vi "HFRR ADV v017 new software.vi"() -> ()   [LabVIEW 2025] (continued)
          tunnel: [w1639] -> w1630
          tunnel: [w1638] -> w1631
          tunnel: w1627 -> [w1637]
          tunnel: w1626 -> [w1636]
          stop <- TRUE stop-if-true
          n1455 = property class="Instr" props=["Serial Settings:Number of Bytes at Serial Port"](reference=w1636, error in=w1637) -> (reference out=w1641:refnum<visa-resource-name>, error out=w1640:errorcluster)  [unwired: 1 out]
          n1456 = VISA Read(VISA resource name=w1641, byte count=u32 50, error in (no error)=w1640) -> (VISA resource name out=w1638:refnum<visa-resource-name>, read buffer=→"UNI READ":string, error out=w1639:errorcluster)  [unwired: 1 out]
          n1457 = Wait (ms)(milliseconds to wait=u32 5) -> ()  [unwired: 1 out]
        }
      }
      frame Error {
        w1656 = u16 0 items=["None", "XON/XOFF", "RTS/CTS", "XON/XOFF & RTS/CTS", "DTR/DSR", "XON/XOFF & DTR/DSR"] ("flow control (0:none)  2")
        w1654 = u16 10 items=["1.0"=10, "1.5"=15, "2.0"=20] ("stop bits 2")
        w1652 = u16 0 items=["None", "Odd", "Even", "Mark", "Space"] ("parity 2")
        w1653 = u32 10000  # timeout (10sec)
        n1458 = VISA Close(VISA resource name=w1648, error in (no error)=w1646) -> (error out=w1649:errorcluster)
        n1459 = local write "Port 1a"(FALSE ("Port 1a")) -> ()
        n1460 = local read "Com Port 1"() -> (w1643:refnum<visa-resource-name>)
        n1461 = call <vilib>:"Clear Errors.vi"("error in (no error)"=w1649) -> ("error out"=w1647:errorcluster)  [unwired: 5 in, 1 out]
        n1462 = call-poly "VISA Configure Serial Port"("VISA resource name"=w1643, "timeout (10sec)"=w1653, "baud rate (9600)"=u32 250000 ("baud rate  2"), "data bits (8)"=u16 8 ("data bits  2"), "parity (0:none)"=w1652, "error in (no error)"=w1647, "stop bits (10: 1 bit)"=w1654, "flow control (0:none)"=w1656) -> ("VISA resource name out"=w1657:refnum<visa-resource-name>, "error out"=w1658:errorcluster)  [unwired: 6 in]
        n1463 = flat-sequence {
          tunnel: w1657 -> [w1660]
          tunnel: w1658 -> [w1659]
          tunnel: [w1660] -> w1650
          tunnel: [w1659] -> w1644
          frame #0 {
            n1464 = Wait (ms)(milliseconds to wait=u32 50) -> ()  [unwired: 1 out]
          }
        }
        "Residual Uno" <- ""
        "Port 1 Error" <- w1644
      }
    }
    n1465 = local read "Quit"() -> (w1605:bool)
    "Error Uno" <- w1610
  }
  n1466 = while {
    stop <- w1671 stop-if-true
    # "V0OLTAGE TO STROKE (peice vise calibration)"
    n1467 = local read "LVDT MIN"() -> (w1662:dbl)
    n1468 = Wait (ms)(milliseconds to wait=u32 10) -> ()  [unwired: 1 out]
    n1469 = local read "LVDT Peak"() -> (w1663:dbl)
    n1470 = formula code="// Dynamic Parameterized Linear Interpolation Node\n// Inputs: vpp_val, voltages (Array), distances (Array)\n// Outputs: stroke\n\nint i = 0;\nint segments = 11; // 12 points make 11 interpolation segments\n\n// 1. Lower Boundary Clamp\nif (vpp_val <= voltages[0]) {\n    stroke = distances[0];\n}\n// 2. Upper Boundary Clamp\nelse if (vpp_val >= voltages[segments]) {\n    stroke = distances[segments];\n}\n// 3. Dynamic Segment Search Loop\nelse {\n    stroke = distances[0]; // Fallback baseline\n    for (i = 0; i < segments; i++) {\n        if (vpp_val >= voltages[i] && vpp_val <= voltages[i+1]) {\n            // Standard linear interpolation formula using array lookups\n            stroke = distances[i] + (vpp_val - voltages[i]) * (distances[i+1] - distances[i]) / (voltages[i+1] - voltages[i]);\n            break; // Segment found, safely exit the loop\n        }\n    }\n}"("vpp_val"=w1663, "voltages"="calibration values", "distances"="STROKE") -> ("stroke"=→"LVDT STROKE":dbl)
    n1471 = local read "Calibration Tare Value"() -> (w1667:dbl)
    n1472 = local read "Calibration Tare"() -> (w1665:bool)
    n1473 = Subtract(x=w1662, y=w1667) -> (x-y=→"LVDT STROKE  Calibration":dbl)
    n1474 = case shown="True" w1665 {
      selector: w1665 -> [_ w1673]
      tunnel: w1662 -> [_ w1674]
      frame False {
      }
      frame True {
        n1475 = Not(x=w1673) -> (.not. x?=w1672:bool)
        n1476 = local write "Calibration Tare"(w1672) -> ()
        "Calibration Tare Value" <- w1674
      }
    }
    n1477 = local read "Quit"() -> (w1671:bool)
  }
  n1478 = while {
    stop <- w1694 stop-if-true
    n1479 = call <vilib>:"High Resolution Polling Wait.vi"("seconds to wait"=0.02) -> ()  [unwired: 10 in, 1 out]
    n1480 = local read "Due read"() -> (w1692:string)
    n1481 = Spreadsheet String To Array(delimiter (Tab)=";", format string="", spreadsheet string=w1692, array type (2D Dbl)=string[] []) -> (array=w1689:string[])
    n1482 = Fract/Exp String To Number(string=w1689) -> (number=w1688:dbl[])  [unwired: 3 in, 1 out]
    n1483 = Index Array(array=w1688) -> (element #1=→"Sample Temperature":dbl, element #2=→"Target Sample Temperature":dbl, element #3=→"Current Duty Cycle":dbl, element #4=→"Ambient Temperature":dbl, element #5=→"Dac Status":dbl, element #6=→"Vpp":dbl, element #7=→"Active Error Code":dbl, element #8=→"Kp":dbl, element #9=→"Ki":dbl, element #10=→"Kd":dbl, element #11=→"SampleRaw":dbl, element #12=→"AmbRaw":dbl)  [unwired: 12 in]
    n1484 = local read "Quit"() -> (w1694:bool)
  }
  n1485 = while {
    shift-right: [w1708] -> w38
    shift-left: _ -> [w1699]
    shift-right: [w1707] -> w37
    shift-left: errorcluster {"status"=FALSE, "code"=0, "source"="Init"} ("error out") -> [w1701]
    tunnel: [w1696] -> w42
    tunnel: [w1706] -> _
    i -> [w1706]
    stop <- w1696 stop-if-true
    n1486 = local read "Com Port 2"() -> (w1700:refnum<visa-resource-name>)
    n1487 = local read "Port 2a"() -> (w1702:bool)
    n1488 = Unbundle(w1701) -> ("status"=→"Port 4":bool)  [unwired: 2 out]
    n1489 = call <vilib>:"High Resolution Polling Wait.vi"("seconds to wait"=0.02) -> ()  [unwired: 10 in, 1 out]
    n1490 = local read "Port 4"() -> (w1703:bool)
    n1491 = Not Equal?(x=w1700, y=w1699) -> (x != y?=w1698:bool)
    n1492 = Or(x=w1703, y=w1702) -> (x .or. y?=w1705:bool)
    n1493 = case shown="False" w1705 {
      frame False {
        w1711 = TRUE ("Visible")
        n1494 = property on="Port 2a" class="Bool (strict)"("Visible"=w1711) -> ()  [unwired: 2 in, 2 out]
        n1495 = property on="Port 4" class="Bool (strict)"("Visible"=w1711) -> ()  [unwired: 2 in, 2 out]
      }
      frame True {
        w1712 = TRUE ("Visible")
        n1496 = property on="Port 2a" class="Bool (strict)"("Visible"=w1712) -> ()  [unwired: 2 in, 2 out]
        n1497 = property on="Port 4" class="Bool (strict)"("Visible"=w1712) -> ()  [unwired: 2 in, 2 out]
      }
    }
    n1498 = case shown="True" w1698 {
      tunnel: [w1709 errorcluster {"status"=TRUE, "code"=0, "source"="Init"} ("error out")] -> w1697
      tunnel: w1701 -> [w1709 _]
      frame False {
      }
      frame True {
      }
    }
    n1499 = case shown="No Error" w1697 {
      selector: w1697 -> [w1725 w1756]
      tunnel: [w1718 w1761] -> w1708
      tunnel: [w1726 w1754] -> w1707
      tunnel: w1699 -> [w1727 w1759]
      frame No Error {
        n1500 = property class="Instr" props=["Serial Settings:Number of Bytes at Serial Port"](reference=w1727, error in=w1725) -> (reference out=w1719:refnum<visa-resource-name>, error out=w1724:errorcluster)  [unwired: 1 out]
        n1501 = while {
          tunnel: [w1735] -> w1720
          tunnel: [w1734] -> w1721
          tunnel: w1724 -> [w1733]
          tunnel: w1719 -> [w1732]
          tunnel: [w1731] -> _
          i -> [w1731]
          stop <- TRUE stop-if-true
          n1502 = property class="Instr" props=["Serial Settings:Number of Bytes at Serial Port"](reference=w1732, error in=w1733) -> (reference out=w1737:refnum<visa-resource-name>, error out=w1736:errorcluster)  [unwired: 1 out]
          n1503 = VISA Read(VISA resource name=w1737, byte count=u32 1000, error in (no error)=w1736) -> (VISA resource name out=w1734:refnum<visa-resource-name>, read buffer=→"Due read":string, error out=w1735:errorcluster)  [unwired: 1 out]
        }
        n1504 = local read "Command"() -> (w1717:string)
        n1505 = call <vilib>:"Trim Whitespace.vi"("string"=w1717) -> ("trimmed string"=w1716:string)  [unwired: 1 in]
        n1506 = Not Equal?(x=w1716, y="") -> (x != y?=w1722:bool)
        n1507 = VISA Flush I/O Buffer(VISA resource name=w1721) -> (VISA resource name out=w1714:refnum<visa-resource-name>, error out=→"error out 10":errorcluster)  [unwired: 2 in]
        n1508 = case shown="True" w1722 {
          tunnel: w1714 -> [w1739 w1744]
          tunnel: [w1739 w1748] -> w1718
          tunnel: w1720 -> [w1738 w1743]
          tunnel: [w1738 w1746] -> w1726
          tunnel: w1716 -> [_ w1742]
          tunnel: [_ w1745] -> _
          frame False {
            # "DATA  WRITE LOOP"
          }
          frame True {
            n1509 = Concatenate Strings(w1742, "\r\n") -> (w1741:string)
            n1510 = VISA Write(VISA resource name=w1744, write buffer=w1741, error in (no error)=w1743) -> (VISA resource name out=w1748:refnum<visa-resource-name>, return count=w1745:u32, error out=w1747:errorcluster)
            n1511 = flat-sequence {
              tunnel: w1747 -> [w1750]
              tunnel: [w1750] -> w1746
              frame #0 {
                n1512 = local write "Command"("" ("Command")) -> ()
                n1513 = Wait (ms)(milliseconds to wait=u32 5) -> ()  [unwired: 1 out]
              }
            }
          }
        }
        "Port 2a" <- TRUE ("Port 2a")
      }
      frame Error {
        w1767 = u16 0 items=["None", "XON/XOFF", "RTS/CTS", "XON/XOFF & RTS/CTS", "DTR/DSR", "XON/XOFF & DTR/DSR"] ("flow control (0:none)  2")
        w1765 = u16 10 items=["1.0"=10, "1.5"=15, "2.0"=20] ("stop bits 2")
        w1763 = u16 0 items=["None", "Odd", "Even", "Mark", "Space"] ("parity 2")
        w1764 = u32 10000  # timeout (10sec)
        n1514 = VISA Clear(VISA resource name=w1759, error in (no error)=w1756) -> (VISA resource name out=w1758:refnum<visa-resource-name>, error out=w1757:errorcluster)
        n1515 = VISA Close(VISA resource name=w1758, error in (no error)=w1757) -> (error out=w1760:errorcluster)
        n1516 = call <vilib>:"Clear Errors.vi"("error in (no error)"=w1760) -> ()  [unwired: 5 in, 2 out]
        n1517 = local write "Port 2a"(FALSE ("Port 2a")) -> ()
        n1518 = local read "Com Port 2"() -> (w1753:refnum<visa-resource-name>)
        "visa due" <- w1753
        n1519 = call-poly "VISA Configure Serial Port"("VISA resource name"=w1753, "timeout (10sec)"=w1764, "baud rate (9600)"=u32 250000 ("baud rate  2"), "data bits (8)"=u16 8 ("data bits  2"), "parity (0:none)"=w1763, "stop bits (10: 1 bit)"=w1765, "flow control (0:none)"=w1767) -> ("VISA resource name out"=w1768:refnum<visa-resource-name>, "error out"=w1769:errorcluster)  [unwired: 7 in]
        n1520 = flat-sequence {
          tunnel: w1768 -> [w1771]
          tunnel: w1769 -> [w1770]
          tunnel: [w1771] -> w1761
          tunnel: [w1770] -> w1754
          frame #0 {
            n1521 = Wait (ms)(milliseconds to wait=u32 50) -> ()  [unwired: 1 out]
          }
        }
        "Residual Due" <- ""
        "Port 2 Error" <- w1754
      }
    }
    n1522 = local read "Quit"() -> (w1696:bool)
    "Error Due" <- w1701
  }
  n1523 = local write "FRICVALZ"(0.0 ("FRICVALZ")) -> ()
  n1524 = property on="RUN" class="Bool (strict)"("Visible"=TRUE) -> ()  [unwired: 2 in, 2 out]
  n1525 = while {
    tunnel: [w1788] -> _
    tunnel: [w1773] -> w55
    i -> [w1788]
    stop <- w1773 stop-if-true
    n1526 = local read "conststatus"() -> (w1777:dbl)
    n1527 = local read "Main Tab"() -> (w1775:T2)
    n1528 = local read "EDIT"() -> (w1794:bool)
    n1529 = local read "Rate"() -> (w1793:dbl)
    n1530 = case shown="True" w1794 {
      tunnel: [FALSE TRUE] -> w1780
      frame False {
      }
      frame True {
      }
    }
    n1531 = property on="Time slide" class="Slide (strict)"("Scale.Range:Maximum"=2500.0) -> ()  [unwired: 2 in, 2 out]
    n1532 = Equal?(x=w1775, y=T27."About" ("Main Tab")) -> (x = y?=w1786:bool)
    n1533 = Equal?(x=w1777, y=0.0) -> (x = y?=w1778:bool)
    n1534 = Divide(x=1.0, y=w1793) -> (x/y=w1789:dbl)
    "Time 2" <- w1789
    n1535 = case shown="True" w1778 {
      frame False {
      }
      frame True {
        # "C:\\WinDucom\\calibrate WO 2391.dcf"
        n1536 = local write "Lan flag"(22) -> ()
        n1537 = local write "conststatus"(10.0 ("rpm value : 2")) -> ()
        n1538 = String To Path(string="C:\\LAB-IQ\\calibrate WO 2465.dcf") -> (path=w1800:path)
        n1539 = Open/Create/Replace File "Open File"(file path (use dialog)=w1800) -> (refnum out=w1798:refnum<file>)  [unwired: 5 in, 2 out]
        n1540 = for {
          N: 23 -> [_]
          tunnel: w1798 -> [w1809]
          i -> [w1803]
          (unwired) TRUE ("line mode (F)")
          n1541 = Read from Text File "Read File"(file (use dialog)=w1809) -> (text=w1808:string)  [unwired: 3 in, 3 out]
          n1542 = Match Pattern(string=w1808, regular expression="]") -> (after substring=w1806:string)  [unwired: 1 in, 3 out]
          n1543 = String Subset(string=w1808, offset (0)=5, length (rest)=10 ("length (rest)")) -> (substring=w1801:string)
          n1544 = Fract/Exp String To Number(string=w1801) -> (number=w1802:dbl)  [unwired: 3 in, 1 out]
          n1545 = Match Pattern(string=w1806, regular expression="-") -> (before substring=w1804:string)  [unwired: 1 in, 3 out]
          n1546 = case shown="4" w1803 {
            tunnel: w1802 -> [w1812 w1813 w1814 w1815 _ _ _ w1820 w1821 _ w1822 w1823 w1824 w1825 w1826 w1827 _ w1828 w1829 _ _ _ _ _]
            tunnel: w1804 -> [_ _ _ _ w1816 w1817 w1818 _ _ _ _ _ _ _ _ _ _ _ _ w1830 w1831 w1832 w1833 _]
            frame 0 {
              n1547 = local write "FRIC. FORCE :"(w1812) -> ()
            }
            frame 1 {
              n1548 = local write "TEMPERATURE :"(w1813) -> ()
            }
            frame 2 {
              n1549 = local write "HUMIDITY:"(w1814) -> ()
            }
            frame 3 {
              n1550 = local write "AIR TEMPERATURE :"(w1815) -> ()
            }
            frame 4 {
              n1551 = local write "Com Port 1"(w1816) -> ()
            }
            frame 5 {
              n1552 = local write "Com Port 2"(w1817) -> ()
              n1553 = local write "visa due"(w1817) -> ()
            }
            frame 6 {
              n1554 = String To Path(string=w1818) -> (path=w1819:path)
              n1555 = local write "File Path"(w1819) -> ()
              "String" <- w1818
            }
            frame 7 {
              n1556 = local write "DISPLACEMENT :"(w1820) -> ()
            }
            frame 8 {
              n1557 = local write "STROKE GAIN :"(w1821) -> ()
            }
            frame 9 {
            }
            frame 10 {
              n1558 = local write "Language Selection"(w1822) -> ()
            }
            frame 11 {
              n1559 = local write "CH-POWER +"(w1823) -> ()
            }
            frame 12 {
              n1560 = local write "CH-POWER -"(w1824) -> ()
            }
            frame 13 {
              n1561 = local write "CH-HEATER"(w1825) -> ()
            }
            frame 14 {
              n1562 = local write "CH-HUMIDITY WET"(w1826) -> ()
            }
            frame 15 {
              n1563 = local write "CH-HUMIDITY DRY"(w1827) -> ()
            }
            frame 16 {
            }
            frame 17 {
              n1564 = local write "AIR TEMP INTERCEPT:"(w1828) -> ()
            }
            frame 18 {
              n1565 = local write "TEMP INTERCEPT:"(w1829) -> ()
            }
            frame 21 {
              n1566 = local write "S.NO"(w1830) -> ()
            }
            frame 22 {
              n1567 = local write "Com Port 3"(w1831) -> ()
            }
            frame 20 {
              n1568 = local write "Camera Port :"(w1832) -> ()
            }
            frame 19 {
              n1569 = local write "C3 :"(w1833) -> ()
            }
            frame 23, Default {
            }
          }
        }
      }
    }
    n1570 = Select(t=u32 2500 ("milliseconds to wait"), s=w1786, f=u32 500 ("milliseconds to wait")) -> (s? t:f=w1784:u32)
    n1571 = Multiply(x=w1789, y=w1784) -> (x*y=w1791:dbl)
    n1572 = property on="Time slide" class="Slide (strict)"("Visible"=w1780) -> ()  [unwired: 2 in, 2 out]
    n1573 = call "Elapsed Time2"("Time Target (s)"=w1791, "Auto Reset"=TRUE) -> ("Time has Elapsed"=w1781:bool)  [unwired: 10 in, 7 out]
    n1574 = case shown="True" w1781 {
      frame False {
      }
      frame True {
        n1575 = stacked-sequence {
          frame #0 {
            # "DATA PROCESSING"
            # "115 mV/N"
            n1576 = local read "Sample Temperature"() -> (w1836:dbl)
            n1577 = local read "RH Numeric:"() -> (w1843:dbl)
            n1578 = local read "HUMIDITY:"() -> (w1844:dbl)
            n1579 = local read "FRICVALZ"() -> (w1855:dbl)
            n1580 = local read "Friction"() -> (w1839:dbl)
            n1581 = Multiply(x=w1843, y=w1844) -> (x*y=→"Humidity ( %RH )" →"Hum" →"Hum 2":dbl)
            n1582 = call <vilib>:"Mean PtByPt.vi"("x"=w1836, "sample length"=100) -> ("mean"=w1835:dbl)  [unwired: 2 in, 1 out]
            "TEMP 2" <- w1835
            "TEMP 3" <- w1835
            n1583 = Subtract(x=w1839, y=w1855) -> (x-y=w1850:dbl)
            "FF 2" <- w1850
            "FF 4" <- w1850
            n1584 = local read "Ambient Temperature"() -> (→"AIR TEMP":dbl)
            n1585 = local read "TEMP"() -> (w1854:dbl)
            n1586 = local write "FF 3"(w1850) -> ()
            n1587 = Compound Arithmetic op=OR("FRICVALZ 4", "FRICVALZ 3", "FRICVALZ 2") -> (w1846:bool)
            n1588 = case shown="True" w1846 {
              tunnel: w1839 -> [_ w1861]
              frame False {
              }
              frame True {
                w1860 = FALSE ("FRICVALZ")
                n1589 = local write "FRICVALZ 3"(w1860) -> ()
                n1590 = local write "FRICVALZ 2"(w1860) -> ()
                n1591 = local write "FRICVALZ 4"(w1860) -> ()
                "FRICVALZ" <- w1861
              }
            }
            n1592 = Not A Number/Path/Refnum?(number/path/refnum=w1854) -> (NaN/Path/Refnum?=w1853:bool)
            n1593 = Not A Number/Path/Refnum?(number/path/refnum=w1850) -> (NaN/Path/Refnum?=w1852:bool)
            n1594 = Divide(x=w1850, y=1.96) -> (x/y=w1847:dbl)
            n1595 = Compound Arithmetic op=OR(w1853, w1852) -> (w1851:bool)
            n1596 = Not A Number/Path/Refnum?(number/path/refnum=w1847) -> (NaN/Path/Refnum?=w1848:bool)
            n1597 = case shown="True" w1851 {
              frame False {
              }
              frame True {
                n1598 = local write "TEMP"(0.0 ("TEMP")) -> ()
                n1599 = local write "FF 2"(0.0 ("FF 2")) -> ()
                n1600 = local write "reinit"(TRUE ("reinit")) -> ()
              }
            }
            n1601 = local write "TEMP"(w1835) -> ()
            n1602 = Select(t=0.0, s=w1848, f=w1847) -> (s? t:f=w1838:dbl)
            "COF 2" <- w1838
            n1603 = local write "COF 3"(w1838) -> ()
          }
        }
      }
    }
    n1604 = Wait (ms)(milliseconds to wait=u32 50) -> ()  [unwired: 1 out]
    n1605 = local read "Quit"() -> (w1773:bool)
    "Rate" <- 2500.0 ("No of Samples")
  }
  n1606 = while {
    tunnel: w58 -> [_]
    tunnel: [w1888] -> _
    tunnel: [w1864] -> w57
    i -> [w1888]
    stop <- w1864 stop-if-true
    # "C:\\LAB-IQ-NXT\\Scar View.exe"
    n1607 = local read "OK Button 16"() -> (w1877:bool)
    n1608 = local read "Main Tab"() -> (w1870:T2)
    n1609 = local read "service 3"() -> (w1871:bool)
    n1610 = local read "OPEN 6"() -> (w1873:bool)
    n1611 = local read "EDIT 2"() -> (w1875:bool)
    n1612 = flat-sequence {
      frame #0 {
        n1613 = local read "SAVE 2"() -> (w2490:bool)
        n1614 = stacked-sequence {
          frame #0 {
            n1615 = local read "EDIT"() -> (w2544:bool)
            n1616 = case shown="True" w2544 {
              tunnel: [u8 2 ("Disabled") u8 0 ("Disabled")] -> _
              frame False {
                w2546 = FALSE
                n1617 = local write "Password"("") -> ()
                n1618 = property on="SrvM CP" class="Bool (strict)"("Visible"=w2546) -> ()  [unwired: 2 in, 2 out]
                n1619 = property on="message" class="Str"("Visible"=w2546) -> ()  [unwired: 2 in, 2 out]
                n1620 = local write "x = y?"(w2546) -> ()
                n1621 = property on="Password" class="Str"("Visible"=w2546) -> ()  [unwired: 2 in, 2 out]
                n1622 = property on="ENTER THE NEW PASSWORD" class="Str"("Visible"=w2546) -> ()  [unwired: 2 in, 2 out]
                n1623 = property on="ENTER CURRENT PASSWORD" class="Str"("Visible"=w2546) -> ()  [unwired: 2 in, 2 out]
                n1624 = local write "SrvM CP"(w2546) -> ()
              }
              frame True {
                w2549 = TRUE
                n1625 = property on="SrvM CP" class="Bool (strict)"("Visible"=w2549) -> ()  [unwired: 2 in, 2 out]
                n1626 = property on="Password" class="Str"("Visible"=w2549) -> ()  [unwired: 2 in, 2 out]
              }
            }
            "dipl pwd" <- "@143$\n" ("dipl pwd")
          }
          frame #1 {
            # "Gain password"
            n1627 = String To Byte Array(string="ENTER CURRENT PASSWORD") -> (unsigned byte array=w2554:u8[])
            n1628 = Search 1D Array(1D array=w2554, element=u8 10) -> (index of element=w2557:i32)  [unwired: 1 in]
            n1629 = Index Array(array=w2554, index=w2557) -> (element=w2553:u8)
            n1630 = Equal?(x=w2553, y=10) -> (x = y?=w2551:bool)
            n1631 = case shown="True" w2551 {
              frame False {
                n1632 = property on="ENTER THE NEW PASSWORD" class="Str"("Visible"=FALSE) -> ()  [unwired: 2 in, 2 out]
              }
              frame True {
                # "password"
                # "change password logic"
                n1633 = local read "ENTER CURRENT PASSWORD"() -> (w2570:string)
                n1634 = local read "dipl pwd"() -> (w2564:string)
                n1635 = String To Byte Array(string=w2570) -> (unsigned byte array=w2572:u8[])
                n1636 = String To Byte Array(string=w2564) -> (unsigned byte array=w2565:u8[])
                n1637 = Array Size(array=w2572) -> (size(s)=w2569:i32)
                n1638 = Array Size(array=w2565) -> (size(s)=w2567:i32)
                n1639 = for {
                  N: w2569 -> [_]
                  tunnel: w2572 -> [w2596]
                  tunnel: [w2594] -> w2573 mode=indexing
                  tunnel: w2569 -> [w2588]
                  i -> [w2589]
                  n1640 = Decrement(x=w2588) -> (x-1=w2586:i32)
                  n1641 = Equal?(x=w2589, y=w2586) -> (x = y?=w2587:bool)
                  n1642 = Index Array(array=w2596, index=w2589) -> (element=w2590:u8)
                  n1643 = Number To Decimal String(number=w2590) -> (decimal integer string=w2595:string)  [unwired: 1 in]
                  n1644 = Select(t="", s=w2587, f="\r") -> (s? t:f=w2592:string)
                  n1645 = Concatenate Strings(w2595, w2592) -> (w2594:string)
                }
                n1646 = for {
                  N: w2567 -> [_]
                  tunnel: w2565 -> [w2584]
                  tunnel: [w2582] -> w2566 mode=indexing
                  tunnel: w2567 -> [w2579]
                  i -> [w2580]
                  n1647 = Decrement(x=w2579) -> (x-1=w2578:i32)
                  n1648 = Equal?(x=w2580, y=w2578) -> (x = y?=w2577:bool)
                  n1649 = Index Array(array=w2584, index=w2580) -> (element=w2583:u8)
                  n1650 = Number To Decimal String(number=w2583) -> (decimal integer string=w2581:string)  [unwired: 1 in]
                  n1651 = Select(t="", s=w2577, f="\r") -> (s? t:f=w2574:string)
                  n1652 = Concatenate Strings(w2581, w2574) -> (w2582:string)
                }
                n1653 = local read "string"() -> (w2571:string)
                n1654 = Concatenate Strings(w2566) -> (w2560:string)
                n1655 = Concatenate Strings(w2571) -> (w2568:string)
                n1656 = Concatenate Strings(w2573) -> (w2561:string)
                n1657 = Equal?(x=w2561, y=w2568) -> (x = y?=w2563:bool)
                n1658 = Equal?(x=w2561, y=w2560) -> (x = y?=w2559:bool)
                n1659 = Or(x=w2563, y=w2559) -> (x .or. y?=w2562:bool)
                n1660 = case shown="True" w2562 {
                  frame False {
                  }
                  frame True {
                    n1661 = property on="ENTER THE NEW PASSWORD" class="Str"("Visible"=TRUE) -> ()  [unwired: 2 in, 2 out]
                  }
                }
              }
            }
          }
          frame #2 {
            n1662 = String To Byte Array(string="ENTER THE NEW PASSWORD") -> (unsigned byte array=w2599:u8[])
            n1663 = Search 1D Array(1D array=w2599, element=u8 10) -> (index of element=w2603:i32)  [unwired: 1 in]
            n1664 = Index Array(array=w2599, index=w2603) -> (element=w2601:u8)
            n1665 = Equal?(x=w2601, y=10) -> (x = y?=w2598:bool)
            n1666 = case shown="False" w2598 {
              frame False {
              }
              frame True {
                n1667 = local write "EDIT"(FALSE) -> ()
                n1668 = local write "SrvM CP"(FALSE) -> ()
                n1669 = local read "ENTER THE NEW PASSWORD"() -> (w2606:string)
                n1670 = String To Byte Array(string=w2606) -> (unsigned byte array=w2611:u8[])
                n1671 = Array Size(array=w2611) -> (size(s)=w2608:i32)
                n1672 = for {
                  N: w2608 -> [_]
                  tunnel: w2611 -> [w2624]
                  tunnel: [w2621] -> w2613 mode=indexing
                  tunnel: w2608 -> [w2616]
                  i -> [w2614]
                  n1673 = Decrement(x=w2616) -> (x-1=w2617:i32)
                  n1674 = Equal?(x=w2614, y=w2617) -> (x = y?=w2618:bool)
                  n1675 = Index Array(array=w2624, index=w2614) -> (element=w2623:u8)
                  n1676 = Number To Decimal String(number=w2623) -> (decimal integer string=w2622:string)  [unwired: 1 in]
                  n1677 = Select(t="", s=w2618, f="\r") -> (s? t:f=w2615:string)
                  n1678 = Concatenate Strings(w2622, w2615) -> (w2621:string)
                }
                n1679 = local read "file path"() -> (w2605:path)
                n1680 = Concatenate Strings(w2613) -> (w2607:string)
                n1681 = Delete(path (use dialog)=w2605) -> (deleted path=w2609:path)  [unwired: 4 in, 2 out]
                n1682 = call <vilib>:"Write Characters To File.vi"("append to file? (new file:F)"=FALSE, "character string"=w2607, "file path (dialog if empty)"=w2609) -> ()  [unwired: 2 in, 1 out]
              }
            }
          }
          frame #3 {
            n1683 = case shown="True" "SrvM CP" {
              frame False {
                w2627 = ""
                n1684 = local write "ENTER CURRENT PASSWORD"(w2627) -> ()
                n1685 = local write "ENTER THE NEW PASSWORD"(w2627) -> ()
                n1686 = property on="ENTER CURRENT PASSWORD" class="Str"("Visible"=FALSE) -> ()  [unwired: 2 in, 2 out]
              }
              frame True {
                n1687 = property on="ENTER THE NEW PASSWORD" class="Str"() -> ("Visible"=w2628:bool)  [unwired: 2 in, 2 out]
                n1688 = Not(x=w2628) -> (.not. x?=w2629:bool)
                n1689 = property on="ENTER CURRENT PASSWORD" class="Str"("Visible"=w2629) -> ()  [unwired: 2 in, 2 out]
              }
            }
          }
          frame #4 {
            n1690 = String To Byte Array(string="Password") -> (unsigned byte array=w2636:u8[])
            n1691 = Search 1D Array(1D array=w2636, element=u8 10) -> (index of element=w2634:i32)  [unwired: 1 in]
            n1692 = Index Array(array=w2636, index=w2634) -> (element=w2635:u8)
            n1693 = Equal?(x=w2635, y=10) -> (x = y?=w2631:bool)
            n1694 = case shown="True" w2631 {
              frame False {
              }
              frame True {
                # "password"
                # "password"
                n1695 = local read "Password"() -> (w2649:string)
                n1696 = String To Byte Array(string=w2649) -> (unsigned byte array=w2652:u8[])
                n1697 = String To Byte Array(string="@143$\n") -> (unsigned byte array=w2638:u8[])
                n1698 = Array Size(array=w2652) -> (size(s)=w2647:i32)
                n1699 = Array Size(array=w2638) -> (size(s)=w2643:i32)
                n1700 = for {
                  N: w2647 -> [_]
                  tunnel: w2652 -> [w2686]
                  tunnel: [w2684] -> w2653 mode=indexing
                  tunnel: w2647 -> [w2681]
                  i -> [w2682]
                  n1701 = Decrement(x=w2681) -> (x-1=w2680:i32)
                  n1702 = Index Array(array=w2686, index=w2682) -> (element=w2685:u8)
                  n1703 = Equal?(x=w2682, y=w2680) -> (x = y?=w2679:bool)
                  n1704 = Number To Decimal String(number=w2685) -> (decimal integer string=w2683:string)  [unwired: 1 in]
                  n1705 = Select(t="", s=w2679, f="\r") -> (s? t:f=w2676:string)
                  n1706 = Concatenate Strings(w2683, w2676) -> (w2684:string)
                }
                n1707 = for {
                  N: w2643 -> [_]
                  tunnel: w2638 -> [w2697]
                  tunnel: [w2695] -> w2641 mode=indexing
                  tunnel: w2643 -> [w2692]
                  i -> [w2693]
                  n1708 = Decrement(x=w2692) -> (x-1=w2691:i32)
                  n1709 = Index Array(array=w2697, index=w2693) -> (element=w2696:u8)
                  n1710 = Equal?(x=w2693, y=w2691) -> (x = y?=w2690:bool)
                  n1711 = Number To Decimal String(number=w2696) -> (decimal integer string=w2694:string)  [unwired: 1 in]
                  n1712 = Select(t="", s=w2690, f="\r") -> (s? t:f=w2687:string)
                  n1713 = Concatenate Strings(w2694, w2687) -> (w2695:string)
                }
                n1714 = local read "file path"() -> (w2637:path)
                n1715 = call <vilib>:"Read Characters From File.vi"("file path (dialog if empty)"=w2637) -> ("character string"=w2651:string)  [unwired: 5 in, 3 out]
                "string" <- w2651
                n1716 = flat-sequence {
                  tunnel: [w2654] -> w2648
                  frame #0 {
                    w2654 = ""
                    n1717 = local write "Password"(w2654) -> ()
                  }
                }
                n1718 = Concatenate Strings(w2641) -> (w2642:string)
                n1719 = Concatenate Strings(w2651) -> (w2650:string)
                n1720 = Concatenate Strings(w2653) -> (w2645:string)
                n1721 = Equal?(x=w2645, y=w2650) -> (x = y?=w2640:bool)
                n1722 = Equal?(x=w2645, y=w2642) -> (x = y?=w2646:bool)
                n1723 = Or(x=w2640, y=w2646) -> (x .or. y?=w2639:bool)
                "x = y?" <- w2639
                n1724 = case shown="True" w2639 {
                  selector: w2639 -> [w2656 _]
                  tunnel: w2648 -> [_ _]
                  frame False {
                    n1725 = And(x=w2656, y=TRUE ("Visible")) -> (x .and. y?=w2657:bool)
                    n1726 = property on="message" class="Str"("Visible"=w2657) -> ()  [unwired: 2 in, 2 out]
                  }
                  frame True {
                    n1727 = control-ref of="This VI"() -> (w2668:refnum<vi>)
                    n1728 = property class="VI"(reference=w2668) -> (reference out=w2659:refnum<vi>, error out=w2663:errorcluster, "Panel"=w2667:refnum<vi>)  [unwired: 1 in]
                    n1729 = property on="message" class="Str"("Visible"=FALSE) -> ()  [unwired: 2 in, 2 out]
                    n1730 = property class="Pnl"(reference=w2667, error in=w2663) -> (reference out=w2661:refnum<vi>, error out=w2664:errorcluster, "Panes[]"=w2666:refnum<vi>[])
                    n1731 = for {
                      tunnel: w2666 -> [w2675] mode=indexing
                      tunnel: T21."Always On" ("Horizontal Scrollbar Visibility") -> [w2674]
                      tunnel: w2664 -> [w2671]
                      tunnel: [w2670] -> w2662
                      n1732 = property class="Pane"(reference=w2675, error in=w2671, "HorizScrollbarVisibility"=w2674) -> (reference out=w2672:refnum<vi>, error out=w2673:errorcluster)
                      n1733 = Close Reference(reference=w2672, error in (no error)=w2673) -> (error out=w2670:errorcluster)
                    }
                    n1734 = Close Reference(reference=w2661, error in (no error)=w2662) -> (error out=w2660:errorcluster)
                    n1735 = Close Reference(reference=w2659, error in (no error)=w2660) -> (error out=→"error out 6":errorcluster)
                  }
                }
              }
            }
          }
        }
        n1736 = local read "x = y?"() -> (w2496:bool)
        n1737 = local read "HUMIDITY: 2"() -> (w2498:dbl)
        n1738 = local read "HUMIDITY:"() -> (w2497:dbl)
        n1739 = property on="Port 2 Error" class="Clust (strict)"("Visible"="EDIT") -> ()  [unwired: 2 in, 2 out]
        n1740 = property on="Port 1 Error" class="Clust (strict)"("Visible"="EDIT") -> ()  [unwired: 2 in, 2 out]
        n1741 = case shown="True" "SrvM CP 2" {
          frame False {
          }
          frame True {
            n1742 = local write "SrvM CP 2"(FALSE ("SrvM CP 2")) -> ()
            n1743 = local read "HUMIDITY: 2"() -> (w2537:dbl)
            n1744 = local read "TEMP INTERCEPT: 2"() -> (w2536:dbl)
            n1745 = local read "DISPLACEMENT : 4"() -> (w2540:dbl)
            n1746 = local read "TEMPERATURE : 2"() -> (w2539:dbl)
            n1747 = local read "STROKE GAIN : 2"() -> (w2541:dbl)
            n1748 = local read "FRIC. FORCE : 2"() -> (w2542:dbl)
            n1749 = local read "AIR TEMP INTERCEPT: 2"() -> (w2535:dbl)
            n1750 = local read "AIR TEMPERATURE : 2"() -> (w2538:dbl)
            n1751 = local write "HUMIDITY:"(w2537) -> ()
            n1752 = local write "AIR TEMP INTERCEPT:"(w2536) -> ()
            n1753 = local write "TEMPERATURE :"(w2539) -> ()
            n1754 = local write "FRIC. FORCE :"(w2542) -> ()
            n1755 = local write "STROKE GAIN :"(w2541) -> ()
            n1756 = local write "DISPLACEMENT :"(w2540) -> ()
            n1757 = local write "AIR TEMPERATURE :"(w2538) -> ()
            n1758 = local write "TEMP INTERCEPT:"(w2535) -> ()
          }
        }
        n1759 = Or(x="SAVE", y=w2490) -> (x .or. y?=w2491:bool)
        n1760 = And(x="EDIT", y=w2496) -> (x .and. y?=w2494:bool)
        n1761 = local read "DISPLACEMENT : 4"() -> (w2507:dbl)
        n1762 = local read "TEMPERATURE : 2"() -> (w2505:dbl)
        n1763 = local read "STROKE GAIN : 2"() -> (w2511:dbl)
        n1764 = local read "DISPLACEMENT :"() -> (w2506:dbl)
        n1765 = local read "FRIC. FORCE : 2"() -> (w2514:dbl)
        n1766 = local read "TEMPERATURE :"() -> (w2503:dbl)
        n1767 = local read "STROKE GAIN :"() -> (w2510:dbl)
        n1768 = local read "FRIC. FORCE :"() -> (w2513:dbl)
        n1769 = case shown="True" w2494 {
          tunnel: [u8 2 ("Disabled") u8 0 ("Disabled")] -> w2493
          tunnel: [w2858 TRUE ("Visible")] -> w2492
          frame False {
            w2858 = FALSE ("Visible")
            n1770 = local write "EDIT 2"(w2858) -> ()
          }
          frame True {
          }
        }
        n1771 = case shown="True" w2491 {
          frame False {
          }
          frame True {
            n1772 = stacked-sequence {
              seq-local: [w2706 _ _] -> [_ w2853 _]
              frame #0 {
                (unwired) i16 5 ("precision (6)")
                # "[CH1]    - FF\n[CH2]   - TEMPERATURE\n[CH3]    - Humidity\n[CH4]    - AIR TEMP\n[CH5]\\- Visa Uno\n[CH6] \\- Visa Due\n[CH7]  \\- file path\n[CH8]   - Displacement Gain\n[CHA]   - Stroke Gain\n[CHB]   - Stroke PID Gain\n[CHC]   -Language Selection\n[CHD]   -Power +\n[CHE]   -Power_\n[CHF]   -Heater\n[CHG]   -Humidity Wet\n[CHH]   -Humidity Dry\n[CHI]   -Integral Time"
                n1773 = local read "Language Selection"() -> (w2754:enum16{"English", "Russian"})
                n1774 = local read "CH-HUMIDITY WET"() -> (w2712:u16)
                n1775 = local read "CH-HUMIDITY DRY"() -> (w2709:u16)
                n1776 = local read "STROKE GAIN :"() -> (w2698:dbl)
                n1777 = local read "CH-POWER +"() -> (w2721:u16)
                n1778 = local read "CH-POWER -"() -> (w2718:u16)
                n1779 = local read "CH-HEATER"() -> (w2715:u16)
                n1780 = local read "AIR TEMPERATURE :"() -> (w2701:dbl)
                n1781 = local read "DISPLACEMENT :"() -> (w2699:dbl)
                n1782 = local read "TEMPERATURE :"() -> (w2702:dbl)
                n1783 = local read "FRIC. FORCE :"() -> (w2703:dbl)
                n1784 = local read "HUMIDITY:"() -> (w2700:dbl)
                n1785 = Path To String(path="File Path") -> (string=w2770:string)
                n1786 = Number To Fractional String(number=w2698, width (-)=i16 10 ("precision (6)"), precision (6)=i16 5) -> (F-format string=w2761:string)  [unwired: 1 in]
                n1787 = Number To Fractional String(number=w2754, width (-)=i16 10 ("precision (6)"), precision (6)=i16 5) -> (F-format string=w2750:string)  [unwired: 1 in]
                n1788 = Number To Fractional String(number=w2721, width (-)=i16 10 ("precision (6)"), precision (6)=i16 5) -> (F-format string=w2744:string)  [unwired: 1 in]
                n1789 = Number To Fractional String(number=w2718, width (-)=i16 10 ("precision (6)"), precision (6)=i16 5) -> (F-format string=w2741:string)  [unwired: 1 in]
                n1790 = Number To Fractional String(number=w2715, width (-)=i16 10 ("precision (6)"), precision (6)=i16 5) -> (F-format string=w2736:string)  [unwired: 1 in]
                n1791 = Number To Fractional String(number=w2712, width (-)=i16 10 ("precision (6)"), precision (6)=i16 5) -> (F-format string=w2733:string)  [unwired: 1 in]
                n1792 = Number To Fractional String(number=w2709, width (-)=i16 10 ("precision (6)"), precision (6)=i16 5) -> (F-format string=w2728:string)  [unwired: 1 in]
                n1793 = local read "Com Port 1"() -> (w2705:refnum<visa-resource-name>)
                n1794 = local read "Com Port 2"() -> (w2704:refnum<visa-resource-name>)
                n1795 = Concatenate Strings(w2770, "\\" ("string")) -> (w2769:string)
                n1796 = Number To Fractional String(number=w2703, width (-)=i16 10 ("precision (6)"), precision (6)=i16 5) -> (F-format string=w2802:string)  [unwired: 1 in]
                n1797 = Number To Fractional String(number=w2702, width (-)=i16 10 ("precision (6)"), precision (6)=i16 5) -> (F-format string=w2801:string)  [unwired: 1 in]
                n1798 = Number To Fractional String(number=w2700, width (-)=i16 10 ("precision (6)"), precision (6)=i16 5) -> (F-format string=w2795:string)  [unwired: 1 in]
                n1799 = Number To Fractional String(number=w2701, width (-)=i16 10 ("precision (6)"), precision (6)=i16 5) -> (F-format string=w2789:string)  [unwired: 1 in]
                n1800 = Number To Fractional String(number=w2699, width (-)=i16 10 ("precision (6)"), precision (6)=i16 5) -> (F-format string=w2762:string)  [unwired: 1 in]
                n1801 = Concatenate Strings("[CHA]" ("string"), w2761, "- Stroke Gain" ("string"), "\r") -> (w2755:string)
                n1802 = Concatenate Strings("[CHC]" ("string"), w2750, "-Language Selection" ("string"), "\r") -> (w2747:string)
                n1803 = Concatenate Strings("[CHD]" ("string"), w2744, "-Power +" ("string"), "\r") -> (w2726:string)
                n1804 = Concatenate Strings("[CHG]" ("string"), w2733, "-Humidity Wet" ("string"), "\r") -> (w2723:string)
                n1805 = Concatenate Strings("[CHH]" ("string"), w2728, "-Humidity Dry" ("string"), "\r") -> (w2722:string)
                n1806 = Concatenate Strings("[CH1]" ("string"), w2802, " - FF" ("string"), "\r") -> (w2800:string)
                n1807 = Concatenate Strings("[CH2]" ("string"), w2801, " - TEMPERATURE" ("string"), "\r") -> (w2799:string)
                n1808 = Concatenate Strings("[CH3]" ("string"), w2795, " - Humidity" ("string"), "\r") -> (w2792:string)
                n1809 = Concatenate Strings("[CH4]" ("string"), w2789, " - AIR TEMP" ("string"), "\r") -> (w2785:string)
                n1810 = Concatenate Strings("[CH5]" ("string"), w2705, "- Visa Uno" ("string"), "\r") -> (w2778:string)
                n1811 = Concatenate Strings("[CH6]" ("string"), w2704, "- Visa Due" ("string"), "\r") -> (w2773:string)
                n1812 = Concatenate Strings("[CH7]" ("string"), w2769, "- file path" ("string"), "\r") -> (w2772:string)
                n1813 = Concatenate Strings("[CH8]" ("string"), w2762, "- Displacement Gain" ("string"), "\r") -> (w2765:string)
                n1814 = Concatenate Strings("[CHE]" ("string"), w2741, "-Power_" ("string"), "\r") -> (w2725:string)
                n1815 = Concatenate Strings("[CHF]" ("string"), w2736, "-Heater" ("string"), "\r") -> (w2724:string)
                n1816 = Concatenate Strings(w2800, w2799, w2792, w2785, w2778, w2773, w2772, w2765, w2755, w2747, w2726, w2725, w2724, w2723, w2722) -> (w2706:string)
                "gain" <- w2706
              }
              frame #1 {
                n1817 = local read "Camera Port :"() -> (w2814:string)
                n1818 = local read "C3 :"() -> (w2822:refnum<visa-resource-name>)
                n1819 = local read "TEMP INTERCEPT:"() -> (w2823:dbl)
                n1820 = local read "AIR TEMP INTERCEPT:"() -> (w2824:dbl)
                n1821 = local read "Com Port 3"() -> (w2825:refnum<visa-resource-name>)
                n1822 = Concatenate Strings("[CH8]" ("string"), w2814, "- Visa Camera" ("string"), "\r") -> (w2813:string)
                n1823 = Concatenate Strings("[CH7]" ("string"), w2822, "- Visa Humidity" ("string"), "\r") -> (w2818:string)
                n1824 = Number To Fractional String(number=w2823, width (-)=i16 10 ("precision (6)"), precision (6)=i16 5) -> (F-format string=w2841:string)  [unwired: 1 in]
                n1825 = Concatenate Strings("[CHL]" ("string"), w2825, "- Visa humid" ("string"), "\r") -> (w2828:string)
                n1826 = Number To Fractional String(number=w2824, width (-)=i16 10 ("precision (6)"), precision (6)=i16 5) -> (F-format string=w2848:string)  [unwired: 1 in]
                n1827 = Concatenate Strings("[CHK]" ("string"), w2841, "-TEMP INTERCEPT" ("string"), "\r") -> (w2837:string)
                n1828 = Concatenate Strings("[SNO]" ("string"), "S.NO", "-" ("string"), "\r") -> (w2833:string)
                n1829 = Concatenate Strings("[CHJ]" ("string"), w2848, "-AIR TEMP INTERCEPT" ("string"), "\r") -> (w2838:string)
                n1830 = String To Path(string="C:\\LAB-IQ\\calibrate WO 2465.dcf") -> (path=w2826:path)
                n1831 = Concatenate Strings(w2853, w2838, w2837, w2833, w2828, w2818, w2813) -> (w2852:string)
                n1832 = call <vilib>:"Write Characters To File.vi"("append to file? (new file:F)"=FALSE, "character string"=w2852, "file path (dialog if empty)"=w2826) -> ()  [unwired: 2 in, 1 out]
              }
              frame #2 {
                n1833 = local write "Lan flag"(0.0 ("Lan flag")) -> ()
                n1834 = local write "conststatus"(0.0 ("rpm value : 2")) -> ()
                n1835 = local write "SAVE"(FALSE ("OK Button 14")) -> ()
                n1836 = local write "SAVE 2"(FALSE ("SAVE 2")) -> ()
              }
            }
          }
        }
        n1837 = Subtract(x=w2498, y=w2497) -> (x-y=w2499:dbl)
        n1838 = local read "AIR TEMPERATURE : 2"() -> (w2502:dbl)
        n1839 = local read "AIR TEMPERATURE :"() -> (w2501:dbl)
        n1840 = Divide(x=w2499, y=w2497) -> (x/y=w2521:dbl)
        n1841 = Subtract(x=w2514, y=w2513) -> (x-y=w2512:dbl)
        n1842 = Subtract(x=w2505, y=w2503) -> (x-y=w2504:dbl)
        n1843 = Subtract(x=w2511, y=w2510) -> (x-y=w2509:dbl)
        n1844 = Subtract(x=w2507, y=w2506) -> (x-y=w2508:dbl)
        n1845 = Subtract(x=w2502, y=w2501) -> (x-y=w2500:dbl)
        n1846 = Divide(x=w2512, y=w2513) -> (x/y=w2532:dbl)
        n1847 = Divide(x=w2504, y=w2503) -> (x/y=w2525:dbl)
        n1848 = Divide(x=w2509, y=w2510) -> (x/y=w2529:dbl)
        n1849 = Divide(x=w2508, y=w2506) -> (x/y=w2528:dbl)
        n1850 = Multiply(x=w2521, y=100.0) -> (x*y=→"HUMIDITY  Calibration Error":dbl)
        n1851 = Divide(x=w2500, y=w2501) -> (x/y=w2524:dbl)
        n1852 = Multiply(x=w2532, y=100.0) -> (x*y=→"FRIC. FORCE Calibration Error":dbl)
        n1853 = Multiply(x=w2525, y=100.0) -> (x*y=→"TEMPERATURE  Calibration Error":dbl)
        n1854 = Multiply(x=w2529, y=100.0) -> (x*y=→"STROKE Calibration Error":dbl)
        n1855 = Multiply(x=w2528, y=100.0) -> (x*y=→"DISPLACEMENT  Calibration Error":dbl)
        n1856 = property on="EDIT 2" class="Bool (strict)"("Visible"=w2492) -> ()  [unwired: 2 in, 2 out]
        n1857 = property on="SAVE" class="Bool (strict)"("Visible"=w2492) -> ()  [unwired: 2 in, 2 out]
        n1858 = property on="SrvM CP" class="Bool (strict)"("Disabled"=w2493) -> ()  [unwired: 2 in, 2 out]
        n1859 = property on="visa due" class="CmbBox"("Disabled"=w2493) -> ()  [unwired: 2 in, 2 out]
        n1860 = property on="File Path" class="Path"("Disabled"=w2493) -> ()  [unwired: 2 in, 2 out]
        n1861 = Multiply(x=w2524, y=100.0) -> (x*y=→"AIR TEMPERATURE  Calibration Error":dbl)
        n1862 = property on="Language Selection" class="Enum (strict)"("Visible"=w2492) -> ()  [unwired: 2 in, 2 out]
        n1863 = property on="Tab Control 7" class="TabCtl (strict)"("Disabled"=w2493) -> ()  [unwired: 2 in, 2 out]
        n1864 = property on="AIR TEMP INTERCEPT:" class="DigNum (strict)"("Disabled"=w2493) -> ()  [unwired: 2 in, 2 out]
        n1865 = property on="CH-POWER -" class="DigNum (strict)"("Disabled"=w2493) -> ()  [unwired: 2 in, 2 out]
        n1866 = property on="CH-POWER +" class="DigNum (strict)"("Disabled"=w2493) -> ()  [unwired: 2 in, 2 out]
        n1867 = property on="AIR TEMPERATURE :" class="DigNum (strict)"("Disabled"=w2493) -> ()  [unwired: 2 in, 2 out]
        n1868 = property on="STROKE GAIN :" class="DigNum (strict)"("Disabled"=w2493) -> ()  [unwired: 2 in, 2 out]
        n1869 = property on="SPEED OUT:" class="DigNum (strict)"("Disabled"=w2493) -> ()  [unwired: 2 in, 2 out]
        n1870 = property on="CH-HUMIDITY DRY" class="DigNum (strict)"("Disabled"=w2493) -> ()  [unwired: 2 in, 2 out]
        n1871 = property on="HUMIDITY:" class="DigNum (strict)"("Disabled"=w2493) -> ()  [unwired: 2 in, 2 out]
        n1872 = property on="CH-HUMIDITY WET" class="DigNum (strict)"("Disabled"=w2493) -> ()  [unwired: 2 in, 2 out]
        n1873 = property on="TEMPERATURE :" class="DigNum (strict)"("Disabled"=w2493) -> ()  [unwired: 2 in, 2 out]
        n1874 = property on="DISPLACEMENT :" class="DigNum (strict)"("Disabled"=w2493) -> ()  [unwired: 2 in, 2 out]
        n1875 = property on="CH-HEATER" class="DigNum (strict)"("Disabled"=w2493) -> ()  [unwired: 2 in, 2 out]
        n1876 = property on="TEMP INTERCEPT:" class="DigNum (strict)"("Disabled"=w2493) -> ()  [unwired: 2 in, 2 out]
        n1877 = property on="FRIC. FORCE :" class="DigNum (strict)"("Disabled"=w2493) -> ()  [unwired: 2 in, 2 out]
      }
    }
    n1878 = local read "RUN"() -> (w1887:bool)
    n1879 = local read "RUN"() -> (w1885:bool)
    n1880 = disable-structure shown="Disabled" {
      disable-tunnel: [w1902 _] -> w1868
      disable-tunnel: [w1901 _] -> w1866
      frame Disabled {
        n1881 = local read "Temperature before test"() -> (w1895:dbl)
        n1882 = local read "Temperature after test"() -> (w1908:dbl)
        n1883 = case shown="True" "Save Results" {
          frame False {
          }
          frame True {
            w1924 = "\r"
            n1884 = local write "Save Results"(FALSE ("OK Button 5")) -> ()
            n1885 = local read "Temperature before test"() -> (w1962:dbl)
            n1886 = local read "Temperature after test"() -> (w1964:dbl)
            n1887 = local read "Humidity before test"() -> (w1961:dbl)
            n1888 = local read "Humidity after test"() -> (w1963:dbl)
            n1889 = local read "WS1.4"() -> (w1968:dbl)
            n1890 = local read "AVP"() -> (w1966:dbl)
            n1891 = Number To Fractional String(number=w1968, width (-)=i16 6, precision (6)=i16 1) -> (F-format string=w1928:string)  [unwired: 1 in]
            n1892 = local read "MWSD"() -> (w1965:dbl)
            n1893 = local read "String"() -> (w1957:string)
            n1894 = local read "FILE"() -> (w1960:string)
            n1895 = local read "HCF"() -> (w1967:dbl)
            n1896 = Number To Fractional String(number=w1961, width (-)=i16 6, precision (6)=i16 1) -> (F-format string=w1953:string)  [unwired: 1 in]
            n1897 = Number To Fractional String(number=w1962, width (-)=i16 6, precision (6)=i16 1) -> (F-format string=w1950:string)  [unwired: 1 in]
            n1898 = Number To Fractional String(number=w1963, width (-)=i16 6, precision (6)=i16 1) -> (F-format string=w1946:string)  [unwired: 1 in]
            n1899 = Number To Fractional String(number=w1964, width (-)=i16 6, precision (6)=i16 1) -> (F-format string=w1942:string)  [unwired: 1 in]
            n1900 = Number To Fractional String(number=w1966, width (-)=i16 6, precision (6)=i16 3) -> (F-format string=w1935:string)  [unwired: 1 in]
            n1901 = Concatenate Strings(w1957, w1960) -> (w1979:string)
            n1902 = Number To Fractional String(number=w1965, width (-)=i16 6, precision (6)=i16 1) -> (F-format string=w1939:string)  [unwired: 1 in]
            n1903 = Number To Fractional String(number=w1967, width (-)=i16 6, precision (6)=i16 2) -> (F-format string=w1933:string)  [unwired: 1 in]
            n1904 = Concatenate Strings("(" ("string"), w1928, ")Microns" ("string")) -> (w1927:string)
            n1905 = local read "REMARKS"() -> (w1959:string)
            "REMARKS 2" <- w1959
            n1906 = Concatenate Strings("(" ("string"), w1953, " ) % RH," ("string")) -> (w1954:string)
            n1907 = Concatenate Strings(w1933, ")" ("string")) -> (w1931:string)
            n1908 = Concatenate Strings("(" ("string"), w1950, ")  Deg C ," ("string")) -> (w1949:string)
            n1909 = Concatenate Strings("(" ("string"), w1946, " ) % RH," ("string")) -> (w1945:string)
            n1910 = Concatenate Strings("(" ("string"), w1942, ")  Deg C ," ("string")) -> (w1941:string)
            n1911 = Concatenate Strings("(" ("string"), w1939, ")  Microns," ("string")) -> (w1938:string)
            n1912 = Concatenate Strings("(" ("string"), w1935, ")  kPa," ("string")) -> (w1925:string)
            n1913 = Concatenate Strings(w1979, ".dwm" ("Substring")) -> (w1977:string)
            n1914 = String To Path(string=w1977) -> (path=w1976:path)
            n1915 = Concatenate Strings(w1959, w1924, " Humidity before test= " ("Substring"), w1954, w1924, " Temperature before test = " ("Substring"), w1949, w1924, " Humidity after test= " ("Substring"), w1945, w1924, "Temperature after test = " ("Substring"), w1941, w1924, "MSD = " ("Substring"), w1938, w1924, "  AVP = " ("Substring"), w1925, w1924, "  HCF                     =( " ("Substring"), w1931, w1924, " WS1.4                  = " ("Substring"), w1927, w1924) -> (w1923:string)
            "data" <- w1923
            n1916 = call <vilib>:"Write Characters To File.vi"("append to file? (new file:F)"=FALSE, "character string"=w1923, "file path (dialog if empty)"=w1976) -> ()  [unwired: 2 in, 1 out]
            n1917 = Match Pattern(string=w1923, regular expression="!") -> (after substring=→"export":string)  [unwired: 1 in, 3 out]
          }
        }
        n1918 = Add(x=231.864, y=w1895) -> (x+y=w1892:dbl)
        n1919 = Add(x=231.864, y=w1908) -> (x+y=w1905:dbl)
        n1920 = Divide(x=1705.984, y=w1892) -> (x/y=w1893:dbl)
        n1921 = Divide(x=1705.984, y=w1905) -> (x/y=w1906:dbl)
        n1922 = local read "Humidity before test"() -> (w1897:dbl)
        n1923 = local read "Humidity after test"() -> (w1910:dbl)
        n1924 = Subtract(x=8.017352 ("y"), y=w1893) -> (x-y=w1919:dbl)
        n1925 = Subtract(x=8.017352 ("y"), y=w1906) -> (x-y=w1913:dbl)
        n1926 = expression code="10**y"(w1919) -> (w1899:dbl)
        n1927 = expression code="10**y"(w1913) -> (w1912:dbl)
        n1928 = Multiply(x=w1897, y=w1899) -> (x*y=w1898:dbl)
        n1929 = Multiply(x=w1910, y=w1912) -> (x*y=w1911:dbl)
        n1930 = Divide(x=w1898, y=750.0) -> (x/y=w1914:dbl)
        n1931 = Divide(x=w1911, y=750.0) -> (x/y=w1915:dbl)
        n1932 = Add(x=w1914, y=w1915) -> (x+y=w1916:dbl)
        n1933 = Divide(x=w1916, y=2.0) -> (x/y=w1918:dbl)
        n1934 = local write "AVP"(w1918) -> ()
        n1935 = Subtract(x=1.4, y=w1918) -> (x-y=w1901:dbl)
        n1936 = local read "HCF"() -> (w1902:dbl)
      }
      frame Enabled {
      }
    }
    n1937 = case shown="True" "EDIT 3" {
      frame False {
      }
      frame True {
        n1938 = local write "EDIT 3"(FALSE ("EDIT 3")) -> ()
        n1939 = local write "Main Tab"(T2."About" ("Main Tab")) -> ()
      }
    }
    n1940 = case shown="False" w1887 {
      frame False {
        n1941 = local read "stopT"() -> (w2865:bool)
        n1942 = case shown="True" w2865 {
          frame False {
          }
          frame True {
            n1943 = local write "stopT"(FALSE) -> ()
          }
        }
      }
      frame True {
        "stopT" <- TRUE
      }
    }
    n1944 = case shown="False" w1885 {
      frame False {
      }
      frame True {
      }
    }
    n1945 = case shown="True" w1875 {
      frame False {
        n1946 = property on="Password 2" class="Str"("Visible"=FALSE) -> ()  [unwired: 2 in, 2 out]
        n1947 = local write "Password 2"("" ("Password")) -> ()
      }
      frame True {
        n1948 = property on="Password 2" class="Str"("Visible"=TRUE) -> ()  [unwired: 2 in, 2 out]
        n1949 = Equal?(x="Password 2", y="HFRR1234") -> (x = y?=w2007:bool)
        n1950 = case shown="True" w2007 {
          tunnel: "Password 2" -> [w2010 _]
          frame False {
            n1951 = String Length(string=w2010) -> (length=w2011:i32)
            n1952 = Greater Than 0?(x=w2011) -> (x > 0?=w2009:bool)
            n1953 = case shown="False" w2009 {
              frame False {
                n1954 = property on="Password 2" class="Str"("Caption.Text"="Password (Advance Setting)") -> ()  [unwired: 2 in, 2 out]
              }
              frame True {
                n1955 = property on="Password 2" class="Str"("Caption.Text"="Incorrect Password!") -> ()  [unwired: 2 in, 2 out]
              }
            }
          }
          frame True {
            n1956 = local write "EDIT 2"(FALSE ("EDIT 2")) -> ()
            n1957 = local write "Password 2"("" ("Password")) -> ()
            n1958 = local write "Main Tab"(T2."Advance" ("Main Tab")) -> ()
            n1959 = local write "Main Dashboard Buttons"(T1."Advance" ("Main Dashboard Buttons")) -> ()
          }
        }
      }
    }
    n1960 = case shown="True" "Prog Uno" {
      frame False {
      }
      frame True {
        n1961 = stacked-sequence {
          frame #0 {
            n1962 = Delete(path (use dialog)=path "C:/LAB-IQ-NXT/UNOCOMPILE.bat" ("working directory")) -> ()  [unwired: 4 in, 3 out]
          }
          frame #1 {
            n1963 = local read "Com Port 1"() -> (w2472:refnum<visa-resource-name>)
            n1964 = Concatenate Strings("cmd.exe /c \"mode " ("command line"), w2472, ":1200,n,8,1\"\n" ("command line")) -> (w2477:string)
            n1965 = Concatenate Strings(w2477, "CD\\\nCD WinDucom\navrdude -C avrdude.conf -v -patmega328p -carduino -P" ("command line"), w2472, " -b115200 -D -Uflash:w:UNO_V20.hex:i\n" ("command line"), "\r") -> (w2479:string)
            "STR" <- w2479
            n1966 = call <vilib>:"Write Characters To File.vi"("append to file? (new file:F)"=FALSE, "character string"=w2479, "file path (dialog if empty)"=path "C:/LAB-IQ/UNOCOMPILE.bat" ("working directory")) -> ()  [unwired: 2 in, 1 out]
          }
          frame #2 {
            n1967 = disable-structure shown="Disabled" {
              frame Disabled {
                w2483 = "cmd.exe  /c \"C:\\LAB-IQ-NXT\\UNOCOMPILE.bat\"" ("string")
                n1968 = local write "Prog Uno"(FALSE ("run minimized? (F)")) -> ()
                n1969 = call <vilib>:"System Exec.vi"("expected output size  (4096)"=u32 65535, "run minimized? (F)"=FALSE, "wait until completion? (T)"=TRUE ("run minimized? (F)"), "working directory"=path "C:/LAB-IQ-NXT", "standard input"=w2483, "command line"=w2483) -> ("error out"=w2482:errorcluster, "standard output"=→"String 42":string)  [unwired: 2 in, 2 out]
                "error out 3" <- w2482
                n1970 = flat-sequence {
                  tunnel: w2482 -> [_]
                  frame #0 {
                  }
                }
              }
              frame Enabled {
              }
            }
          }
        }
      }
    }
    n1971 = case shown="\"ISO 12156\"" "TEST STANDARD" {
      tunnel: [2.0 ("Set Temp") 0.0 ("Set Temp") 2.0 ("Set Temp") 0.0 ("Set Temp")] -> w1876
      frame "ASTM D6079", Default {
        w2429 = 50.0 ("Hz")
        w2430 = 53.0 ("Set Rh")
        w2432 = 1.0 ("Set Strk")
        w2431 = 60.0 ("Set Temp")
        # "astm hide"
        n1972 = local write "NORMAL LOAD"(200.0 ("NORMAL LOAD")) -> ()
        n1973 = local write "Set Strk"(w2432) -> ()
        n1974 = local write "Set Hz"(w2429) -> ()
        n1975 = local write "Set Temp"(w2431) -> ()
        n1976 = local write "Set Rh"(w2430) -> ()
        n1977 = local write "test time"(75.0 ("test time")) -> ()
        n1978 = local write "Set Stroke:"(w2432) -> ()
        n1979 = local write "Set Humidity:"(w2430) -> ()
        n1980 = local write "Set Frequency:"(w2429) -> ()
        n1981 = local write "Set Temperature:"(w2431) -> ()
        "Test Standard" <- "ASTM D6079" ("Test Standard 2")
      }
      frame "ISO 12156" {
        n1982 = local write "Set Strk"(1.0 ("Set Strk")) -> ()
        n1983 = local write "NORMAL LOAD"(200.0 ("NORMAL LOAD")) -> ()
        n1984 = local write "Set Temp"(60.0 ("Set Temp")) -> ()
        n1985 = local write "test time"(75.0 ("test time")) -> ()
        n1986 = local write "Set Hz"(50.0 ("Hz")) -> ()
        n1987 = local write "Set Rh"(53.0 ("Set Rh")) -> ()
      }
      frame "CEC F-096-A-06" {
        n1988 = local write "Set Strk"(1.0 ("Set Strk")) -> ()
        n1989 = local write "NORMAL LOAD"(200.0 ("NORMAL LOAD")) -> ()
        n1990 = local write "Set Temp"(60.0 ("Set Temp")) -> ()
        n1991 = local write "test time"(75.0 ("test time")) -> ()
        n1992 = local write "Set Hz"(50.0 ("Hz")) -> ()
        n1993 = local write "Set Rh"(53.0 ("Set Rh")) -> ()
      }
      frame "Custom" {
      }
    }
    n1994 = case shown="True" "Prog Due" {
      frame False {
      }
      frame True {
        n1995 = stacked-sequence {
          frame #0 {
            n1996 = Delete(path (use dialog)=path "C:/LAB-IQ/DUECOMPILE.bat" ("working directory")) -> ()  [unwired: 4 in, 3 out]
          }
          frame #1 {
            n1997 = disable-structure shown="Disabled" {
              frame Disabled {
                n1998 = local read "visa due"() -> (w2454:string)
                n1999 = Concatenate Strings("cmd.exe /c \"mode " ("command line"), w2454, ":1200,n,8,1\"\n" ("command line")) -> (w2459:string)
                n2000 = Concatenate Strings(w2459, "CD\\\nCD WinDucom\nTIMEOUT 1\n bossac.exe -i -d --port=" ("command line"), w2454, " -U false -e -w -v -b DUE.bin -R\n" ("command line"), "\r") -> (w2461:string)
                "concatenated string 2" <- w2461
                n2001 = call <vilib>:"Write Characters To File.vi"("append to file? (new file:F)"=FALSE, "character string"=w2461, "file path (dialog if empty)"=path "C:/LAB-IQ-NXT/DUECOMPILE.bat" ("working directory")) -> ()  [unwired: 2 in, 1 out]
              }
              frame Enabled {
              }
            }
          }
          frame #2 {
            # "C:\\LAB-IQ-NXT\\DUECOMPILE.bat"
            n2002 = disable-structure shown="Disabled" {
              frame Disabled {
                w2466 = "cmd.exe  /c \"C:\\LAB-IQ-NXT\\DUECOMPILE.bat\"" ("string")
                n2003 = call <vilib>:"System Exec.vi"("expected output size  (4096)"=u32 65535, "run minimized? (F)"=FALSE, "wait until completion? (T)"=TRUE ("run minimized? (F)"), "working directory"=path "C:/LAB-IQ-NXT", "standard input"=w2466, "command line"=w2466) -> ("error out"=w2465:errorcluster, "standard output"=→"String 44":string)  [unwired: 2 in, 2 out]
                "error out 4" <- w2465
                n2004 = flat-sequence {
                  tunnel: w2465 -> [_]
                  frame #0 {
                  }
                }
              }
              frame Enabled {
              }
            }
            n2005 = local write "Prog Due"(FALSE ("Prog Due")) -> ()
          }
        }
      }
    }
    n2006 = Or(x=w1873, y=w1871) -> (x .or. y?=w1872:bool)
    n2007 = case shown="\"About\"" w1870 {
      tunnel: [T27."Acquire" ("Main Tab") T27."Compare Files" ("Main Tab") T27."About" ("Main Tab")] -> w1883
      frame "Acquire", Default {
      }
      frame "Compare Files" {
      }
      frame "About" {
      }
    }
    n2008 = Or(x=w1877, y="OPEN") -> (x .or. y?=w1878:bool)
    n2009 = case shown="True" w1878 {
      tunnel: w1877 -> [_ w2018]
      frame False {
      }
      frame True {
        n2010 = stacked-sequence {
          tunnel: w2018 -> [_ w2085 _ _]
          frame #0 {
            w2034 = "  " ("String 6")
            n2011 = local write "OPEN"(FALSE ("open")) -> ()
            n2012 = local read "string1 2"() -> (w2022:string)
            n2013 = local read "string1 3"() -> (w2021:string)
            n2014 = local read "string1 4"() -> (w2020:string)
            n2015 = property on="OPEN" class="Bool (strict)"("Visible"=FALSE) -> ()  [unwired: 2 in, 2 out]
            n2016 = local write "String 6"(w2034) -> ()
            n2017 = local write "String 7"(w2034) -> ()
            n2018 = local write "String 8"(w2034) -> ()
            n2019 = local write "String 12"(w2034) -> ()
            n2020 = local read "OK Button 16"() -> (w2019:bool)
